vi "MBW_Test.vi"() -> ()   [LabVIEW 2009]
uses:
  <vilib>/Instr/_visa.llb/VISA Configure Serial Port (Instr).vi
panel:
  out "error out":errorcluster
  in  "milliseconds to wait":u32=1
  out "Reply":string
  in  "Command":string
  in  "Com Port":refnum<visa-resource-name>
  in  "Send":bool
  in  "stop":bool
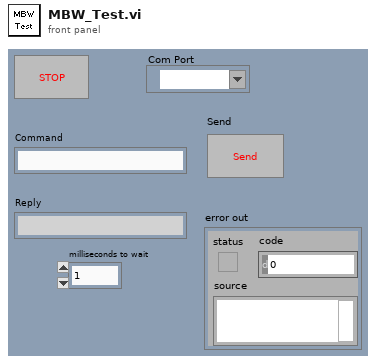
[diagram p1: front panel]
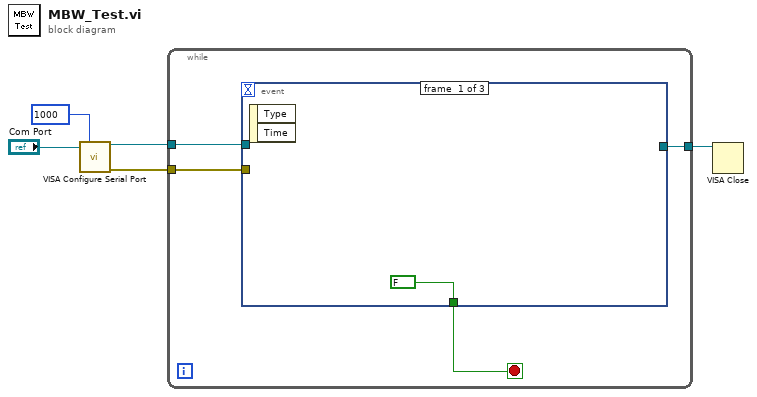
[diagram p0: block diagram]
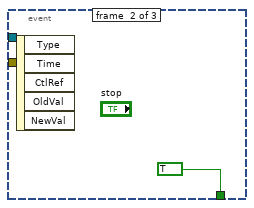
[diagram p2: hidden frame]
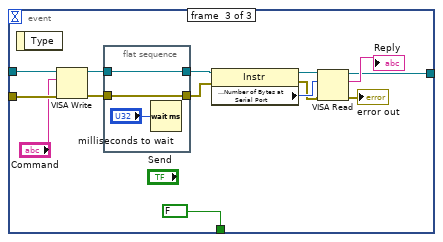
[diagram p3: hidden frame]
diagram:
  n1 = call-poly "VISA Configure Serial Port"("VISA resource name"="Com Port", "timeout (10sec)"=u32 1000) -> ("VISA resource name out"=w4:refnum<visa-resource-name>, "error out"=w2:errorcluster)  [unwired: 12 in]
  n2 = while {
    tunnel: w4 -> [w8]
    tunnel: w2 -> [w7]
    tunnel: [w6] -> w1
    stop <- w9 stop-if-true
    n3 = event shown="[2] \"Send\": Value Change" {
      selector: _ -> [_ _ _]
      dyn-events: _ -> [_ _ _]
      timeout: _ -> [_ _ _]
      tunnel: [FALSE TRUE FALSE] -> w9
      tunnel: w8 -> [_ _ w22]
      tunnel: w7 -> [_ _ w21]
      tunnel: [_ _ w12] -> w6
      event #0 {
        n4 = event-data() -> ()  [unwired: 1 in, 2 out]
      }
      event #1 {
        n5 = event-data() -> ()  [unwired: 1 in, 5 out]
      }
      event #2 {
        n6 = event-data() -> ()  [unwired: 1 in, 1 out]
        n7 = VISA Write(VISA resource name=w22, write buffer="Command", error in (no error)=w21) -> (VISA resource name out=w20:refnum<visa-resource-name>, error out=w18:errorcluster)  [unwired: 1 out]
        n8 = flat-sequence {
          tunnel: w20 -> [w27]
          tunnel: [w27] -> w19
          tunnel: w18 -> [w26]
          tunnel: [w26] -> w17
          frame #0 {
            n9 = Wait (ms)(milliseconds to wait="milliseconds to wait") -> ()  [unwired: 1 out]
          }
        }
        n10 = property class="Instr"(reference=w19, error in=w17) -> (reference out=w24:refnum<visa-resource-name>, error out=w16:errorcluster, "Serial Settings:Number of Bytes at Serial Port"=w23:u32)
        n11 = VISA Read(VISA resource name=w24, byte count=w23, error in (no error)=w16) -> (VISA resource name out=w12:refnum<visa-resource-name>, read buffer=→"Reply":string, error out=→"error out":errorcluster)  [unwired: 1 out]
      }
    }
  }
  n12 = VISA Close(VISA resource name=w1) -> ()  [unwired: 1 in, 1 out]
